vi "getWavesPath.vi"(8 "error in (no error)":errorcluster, 11 "FileSystem.lvclass in":refnum<class "FileSystem.lvclass">) -> (0 "error out":errorcluster, 2 "Waves":path, 3 "FileSystem.lvclass out":refnum<class "FileSystem.lvclass">)   [LabVIEW 2009, in "Tools.lvlib" / "Filing.lvlib" / "FileSystem.lvclass"]
uses:
  FileSystem.lvclass
  FileSystem.lvclass/FileSystem.ctl
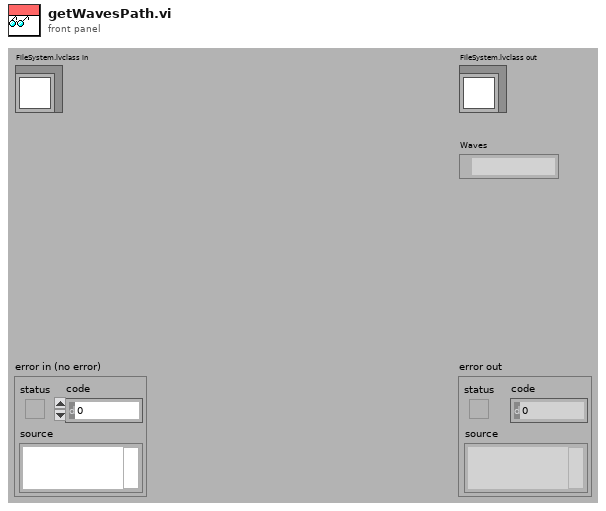
[diagram p1: front panel]
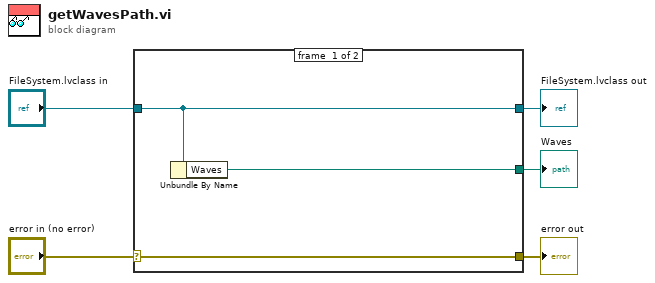
[diagram p0: block diagram]
diagram:
  n1 = case shown="No Error" "error in (no error)" {
    selector: "error in (no error)" -> [w8 w9]
    tunnel: [w8 w9] -> w4
    tunnel: [w7 w10] -> w2
    tunnel: "FileSystem.lvclass in" -> [w7 w10]
    tunnel: [w6 _] -> w1
    frame #0 {
      n2 = Unbundle By Name(w7) -> ("Waves"=w6:path)
    }
    frame #1 {
    }
  }
  "error out" <- w4
  "FileSystem.lvclass out" <- w2
  "Waves" <- w1
